vi "_template_Unmarshal.vi"   [LabVIEW 2019]
uses:
  <vilib>/LabVIEW Open Source Project/OpenSerializer/Serializer/Serializer.lvclass
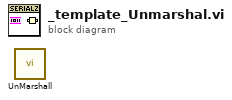
[diagram p0: block diagram]
diagram:
  n1 = call <vilib>:"UnMarshall.vi"() -> ()  [unwired: 9 in, 3 out]
